vi "Query Device Settings.vi"(8 "error in (no error)":errorcluster, 11 "VISA resource name":refnum<visa-resource-name>) -> (0 "error out":errorcluster, 2 "Current Device Setting":T1, 3 "VISA resource name out":refnum<visa-resource-name>)   [LabVIEW 2011, in "Ocean Server OS4000.lvlib"]
doc: "Obtains Compass Setting."
uses:
  Ocean Server OS4000.lvlib
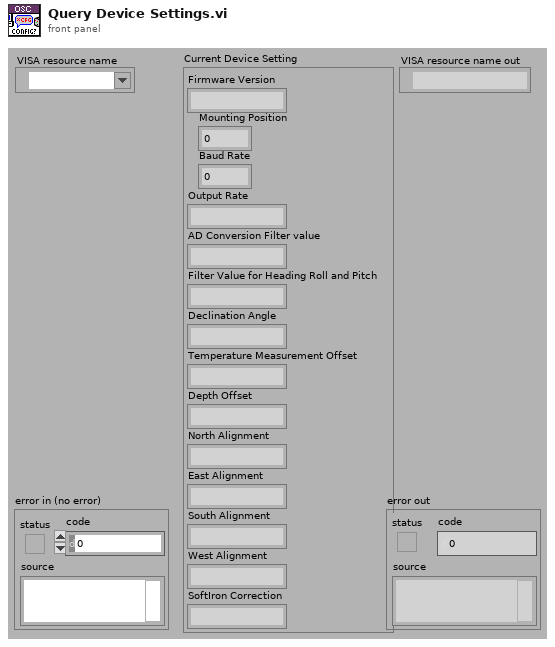
[diagram p1: front panel]
types:
  T1 = cluster{"Firmware Version":string, "Mounting Position":u16, "Baud Rate":u16, "Output Rate":string, "AD Conversion Filter value":string, "Filter Value for Heading Roll and Pitch":string, "Declination Angle":string, "Temperature Measurement Offset":string, "Depth Offset":string, "North Alignment":string, "East Alignment":string, "South Alignment":string, "West Alignment":string, "SoftIron Correction":string}
  T2 = cluster{"Firmare Version":string, "Mounting Position":u16, "Baud Rate":u16, "Output Rate":string, "AD Conversion Filter value":string, "Filter Value for Heading Roll and Pitch":string, "Declination Angle":string, "Temperature Measurement Offset":string, "Depth Offset":string, "North Alignment":string, "East Alignment":string, "South Alignment":string, "West Alignment":string, "SoftIron Correction":string}
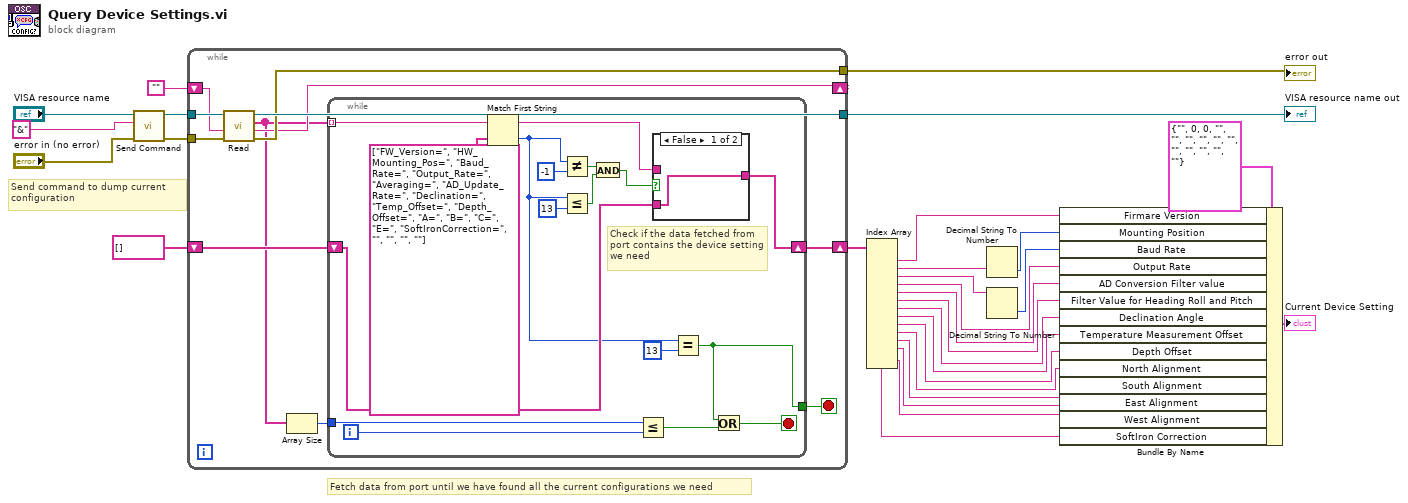
[diagram p0: block diagram]
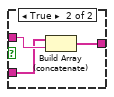
[diagram p2: hidden frame]
diagram:
  # "Fetch data from port until we have found all the current configurations we need"
  # "Send command to dump current\nconfiguration"
  n1 = call "Send Command.vi"("error in (no error)"="error in (no error)", "Message"="&", "VISA resource name"="VISA resource name") -> ("error out"=w6:errorcluster, "VISA resource out"=w25:refnum<visa-resource-name>)  [unwired: 7 in]
  n2 = while {
    tunnel: w25 -> [w39]
    shift-right: [w32] -> w22
    shift-left: string[] [] ("array") -> [w33]
    tunnel: [w38] -> w7
    tunnel: w6 -> [w37]
    tunnel: [w36] -> w5
    shift-right: [w35] -> _
    shift-left: "" ("Remaining Sentence") -> [w34]
    stop <- w31 stop-if-true
    n3 = call "Read.vi"("error in (no error)"=w37, "Text to prepend to sentence"=w34, "VISA resource name"=w39) -> ("error out"=w36:errorcluster, "Remaining Sentence"=w35:string, "Ocean Server Sentences"=w30:string[], "VISA resource name out"=w38:refnum<visa-resource-name>)  [unwired: 5 in]
    n4 = Array Size(array=w30) -> (size(s)=w29:i32)
    n5 = while {
      tunnel: w30 -> [w55] mode=indexing
      shift-right: [w45] -> w32
      shift-left: w33 -> [w53]
      tunnel: [w40] -> w31
      tunnel: w29 -> [w42]
      i -> [w43]
      stop <- w44 stop-if-true
      # "Check if the data fetched from port contains the device setting we need"
      n6 = Match First String(2:string[] ["FW_Version=", "HW_Mounting_Pos=", "Baud_Rate=", "Output_Rate=", "Averaging=", "AD_Update_Rate=", "Declination=", "Temp_Offset=", "Depth_Offset=", "A=", "B=", "C=", "E=", "SoftIronCorrection=", "", "", "", ""], 3:w55) -> (0:w50:i32, 1:w54:string)
      n7 = Not Equal?(x=w50, y=-1) -> (x != y?=w47:bool)
      n8 = Less Or Equal?(x=w50, y=13) -> (x <= y?=w48:bool)
      n9 = And(x=w47, y=w48) -> (x .and. y?=w46:bool)
      n10 = Less Or Equal?(x=w42, y=w43) -> (x <= y?=w41:bool)
      n11 = case shown="False" w46 {
        tunnel: w54 -> [_ w60]
        tunnel: w53 -> [w57 w59]
        tunnel: [w57 w58] -> w45
        frame False {
        }
        frame True {
          n12 = Build Array (concatenate)(w59, w60) -> (w58:string[])
        }
      }
      n13 = Equal?(x=w50, y=13) -> (x = y?=w40:bool)
      n14 = Or(x=w40, y=w41) -> (x .or. y?=w44:bool)
    }
  }
  "VISA resource name out" <- w7
  "error out" <- w5
  n15 = Index Array(array=w22) -> (element #1=w1:string, element #2=w21:string, element #3=w19:string, element #4=w17:string, element #5=w16:string, element #6=w15:string, element #7=w14:string, element #8=w13:string, element #9=w12:string, element #10=w11:string, element #11=w10:string, element #12=w9:string, element #13=w2:string, element #14=w3:string)  [unwired: 14 in]
  n16 = Decimal String To Number(string=w21) -> (number=w20:i32)  [unwired: 2 in, 1 out]
  n17 = Decimal String To Number(string=w19) -> (number=w18:i32)  [unwired: 2 in, 1 out]
  n18 = Bundle By Name(cluster=T2 {"Firmare Version"="", "Mounting Position"=0, "Baud Rate"=0, "Output Rate"="", "AD Conversion Filter value"="", "Filter Value for Heading Roll and Pitch"="", "Declination Angle"="", "Temperature Measurement Offset"="", "Depth Offset"="", "North Alignment"="", "East Alignment"="", "South Alignment"="", "West Alignment"="", "SoftIron Correction"=""} ("Data"), "Firmare Version"=w1, "Mounting Position"=w20, "Baud Rate"=w18, "Output Rate"=w17, "AD Conversion Filter value"=w16, "Filter Value for Heading Roll and Pitch"=w15, "Declination Angle"=w14, "Temperature Measurement Offset"=w13, "Depth Offset"=w12, "North Alignment"=w11, "South Alignment"=w10, "East Alignment"=w9, "West Alignment"=w2, "SoftIron Correction"=w3) -> (→"Current Device Setting":T2)
